vi "fail display1.vi"(1 "P/F":bool[](array[boolean]), 2 "yellow":bool, 3 "Multipart board":cluster{"Row":i32, "Colum":i32}={"Row"=8, "Colum"=4}, 4 "内容区域边界":T1, 5 "Tbl引用句柄":refnum<vi>) -> ()   [LabVIEW 2018]
uses:
  <vilib>/Utility/miscctls.llb/LVBoundsTypeDef.ctl
  <vilib>/Utility/miscctls.llb/LVRowAndColumnTypeDef.ctl
panel:
  out "引用输出":refnum<vi>
  in  "Pass/Fail Dispaly":string[][](table)
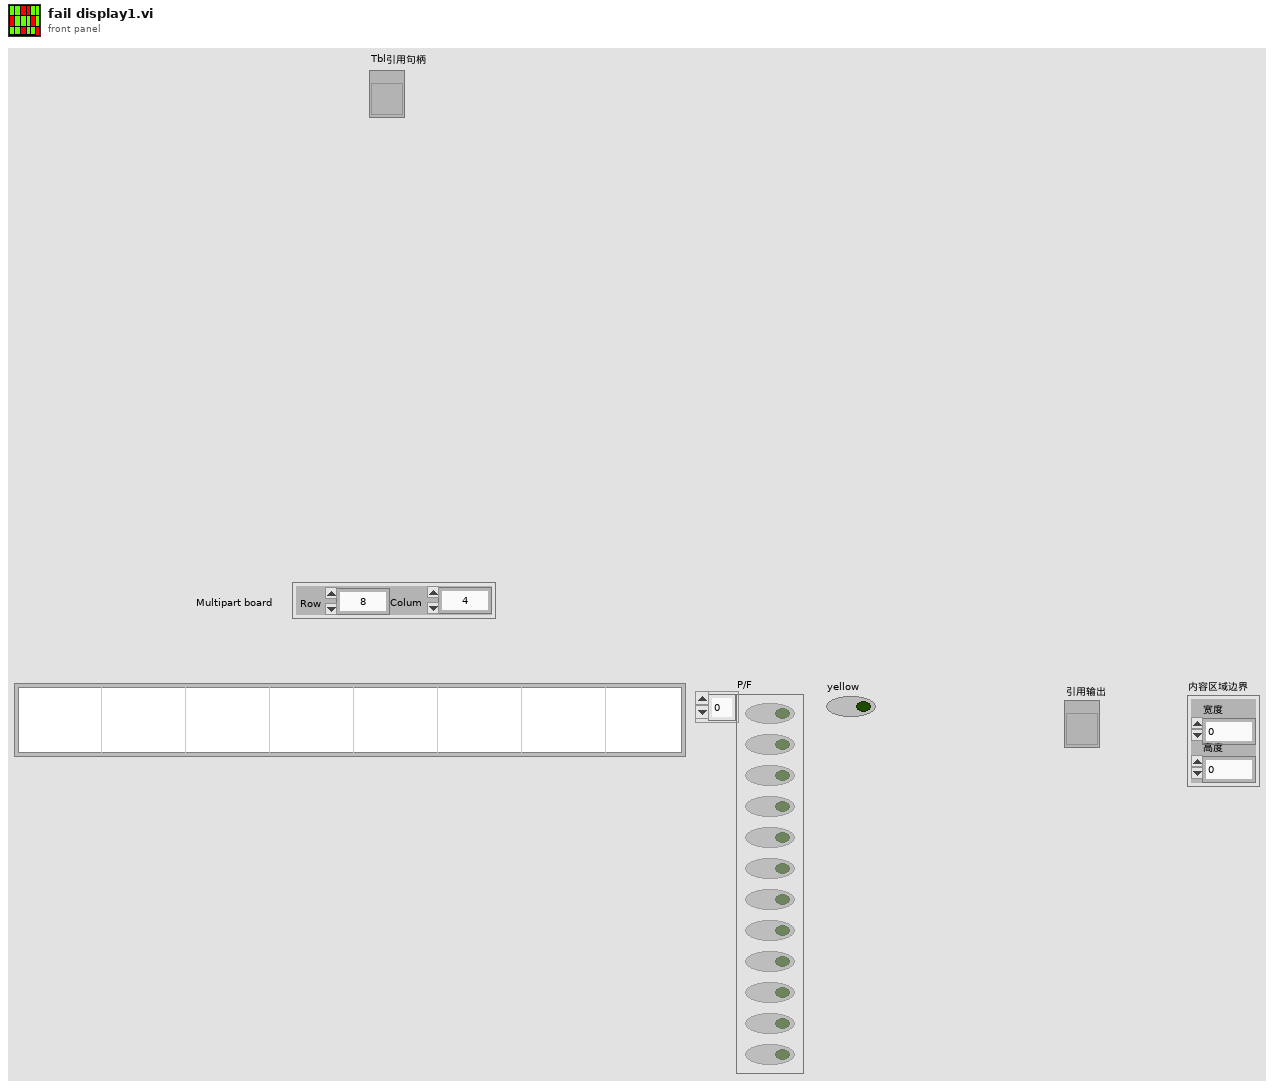
[diagram p1: front panel]
types:
  T1 = typedef "LVBoundsTypeDef.ctl" = cluster{"Width":u32, "Height":u32}
  T2 = typedef "LVRowAndColumnTypeDef.ctl" = cluster{"Row":i32, "Column":i32}
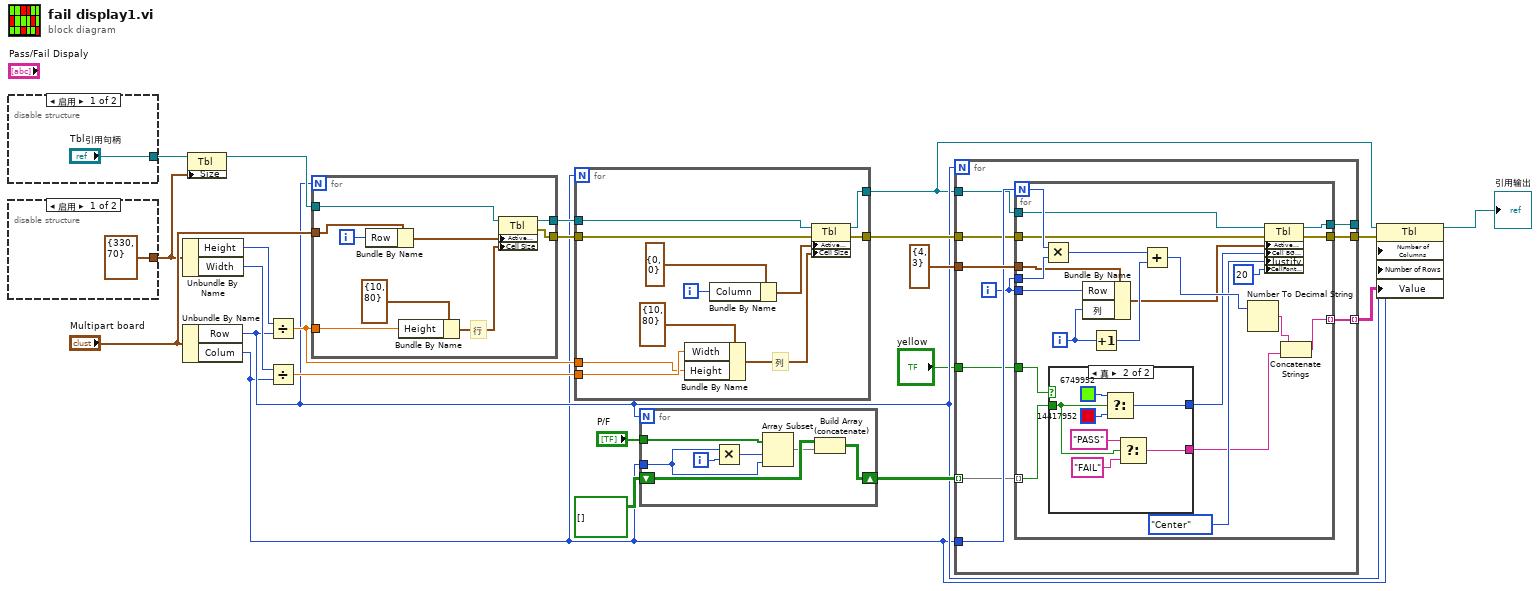
[diagram p0: block diagram]
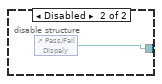
[diagram p2: hidden frame]
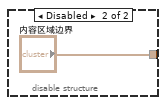
[diagram p3: hidden frame]
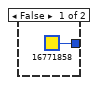
[diagram p4: hidden frame]
diagram:
  n1 = disable-structure shown="启用" {
    disable-tunnel: ["Tbl引用句柄" w24] -> w4
    frame Enabled {
    }
    frame Disabled {
      n2 = control-ref of="Pass/Fail Dispaly"() -> (w24:refnum<vi>)
    }
  }
  n3 = disable-structure shown="启用" {
    disable-tunnel: [T1 {"Width"=330, "Height"=70} ("大小") "内容区域边界"] -> w7
    frame Enabled {
    }
    frame Disabled {
    }
  }
  n4 = Unbundle By Name(w7) -> ("Height"=w18:u32, "Width"=w19:u32)
  n5 = Unbundle By Name("Multipart board") -> ("Row"=w9:i32, "Colum"=w8:i32)
  n6 = property class="Tbl"(reference=w4, "Size"=w7) -> (reference out=w11:refnum<vi>)  [unwired: 1 in, 1 out]
  n7 = Divide(x=w18, y=w9) -> (x/y=w21:dbl)
  n8 = Divide(x=w19, y=w8) -> (x/y=w20:dbl)
  n9 = for {
    N: w9 -> [_]
    tunnel: w21 -> [w34]
    tunnel: "Multipart board" -> [w32]
    tunnel: w11 -> [w31]
    tunnel: [w29] -> w13
    tunnel: [w28] -> w12
    i -> [w33]
    # "行"
    n10 = Bundle By Name(cluster=w32, "Row"=w33) -> (w27:cluster{"Row":i32, "Colum":i32})
    n11 = Bundle By Name(cluster=T1 {"Width"=10, "Height"=80} ("活动单元格:单元格大小"), "Height"=w34) -> (w30:T1)
    n12 = property class="Tbl"(reference=w31, "Active Cell"=w27, "Cell Size"=w30) -> (reference out=w28:refnum<vi>, error out=w29:errorcluster)  [unwired: 1 in]
  }
  n13 = for {
    N: w8 -> [_]
    tunnel: w20 -> [w43]
    tunnel: w21 -> [w42]
    tunnel: w13 -> [w40]
    tunnel: w12 -> [w41]
    tunnel: [w37] -> w3
    tunnel: [w36] -> w10
    i -> [w46]
    # "列"
    n14 = Bundle By Name(cluster=T1 {"Width"=10, "Height"=80} ("活动单元格:单元格大小"), "Width"=w43, "Height"=w42) -> (w38:T1)
    n15 = Bundle By Name(cluster=T2 {"Row"=0, "Column"=0} ("活动单元格:活动单元格"), "Column"=w46) -> (w39:T2)
    n16 = property class="Tbl"(reference=w41, error in=w40, "Active Cell"=w39, "Cell Size"=w38) -> (reference out=w37:refnum<vi>, error out=w36:errorcluster)
  }
  n17 = for {
    N: w9 -> [_]
    shift-right: [w51] -> w16
    shift-left: bool[][] [] ("添加的数组 2") -> [w52]
    tunnel: "P/F" -> [w53]
    tunnel: w8 -> [w47]
    i -> [w49]
    n18 = Multiply(x=w47, y=w49) -> (x*y=w48:i32)
    n19 = Array Subset(array=w53, index=w48, length=w47) -> (w50:bool[])
    n20 = Build Array (concatenate)(w52, w50) -> (w51:bool[][])
  }
  n21 = for {
    N: w9 -> [_]
    tunnel: w8 -> [w62]
    tunnel: cluster{"Row":i32, "列":i32} {"Row"=4, "列"=3} ("多联板 2") -> [w63]
    tunnel: w16 -> [w60] mode=indexing
    tunnel: w10 -> [w56]
    tunnel: w3 -> [w59]
    tunnel: [w58] -> _
    tunnel: [w57] -> w6 mode=indexing
    tunnel: [w55] -> w5
    tunnel: "yellow" -> [w54]
    i -> [w61]
    n22 = for {
      N: w62 -> [w77]
      tunnel: w61 -> [w84]
      tunnel: w63 -> [w81]
      tunnel: w61 -> [w80]
      tunnel: w60 -> [w79] mode=indexing
      tunnel: w59 -> [w75]
      tunnel: [w74] -> w58
      tunnel: [w65] -> w57 mode=indexing
      tunnel: w56 -> [w69]
      tunnel: [w68] -> w55
      tunnel: w54 -> [w67]
      i -> [w78]
      n23 = Multiply(x=w77, y=w84) -> (x*y=w83:i32)
      n24 = case shown="真" w67 {
        tunnel: w79 -> [_ w87]
        tunnel: [u32 16771858 w90] -> w73
        tunnel: [_ w86] -> w64
        frame False {
        }
        frame True {
          n25 = Select(t=u32 6749952, s=w87, f=u32 14417952) -> (s? t:f=w90:u32)
          n26 = Select(t="PASS", s=w87, f="FAIL") -> (s? t:f=w86:string)
        }
      }
      n27 = Bundle By Name(cluster=w81, "Row"=w80, "列"=w78) -> (w72:cluster{"Row":i32, "列":i32})
      n28 = Increment(x=w78) -> (x+1=w82:i32)
      n29 = Add(x=w83, y=w82) -> (x+y=w76:i32)
      n30 = Number To Decimal String(number=w76) -> (decimal integer string=w66:string)  [unwired: 1 out]
      n31 = property class="Tbl"(reference=w75, error in=w69, "Active Cell"=w72, "Cell BG Color"=w73, "Justify"=enum16{"Left", "Center", "Right"}."Center" ("活动单元格:单元格对齐"), "CellFontSize"=u32 20 ("活动单元格:单元格字体:字号")) -> (reference out=w74:refnum<vi>, error out=w68:errorcluster)
      n32 = Concatenate Strings(w66, w64) -> (w65:string)
    }
  }
  n33 = property class="Tbl"(reference=w3, error in=w5, "Number of Columns"=w8, "Number of Rows"=w9, "Value"=w6) -> (reference out=→"引用输出":refnum<vi>)  [unwired: 1 out]
